vi "Stack Management.vi"(0 "Suck":bool) -> (1 "IsSucking?":bool, 2 "Full Stack (4 discs in)":bool)   [LabVIEW 2012]
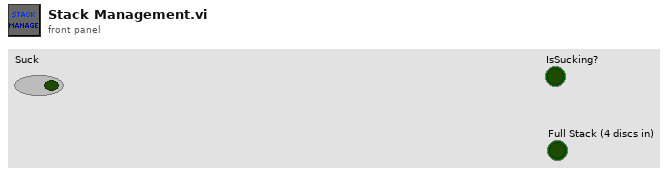
[diagram p1: front panel]
types:
  T1 = typedef "WPI_MotorControlDeviceRef.ctl" = cluster{"DeviceStatus":errorcluster, "Type":enum16{"PWM", "CAN"}, "PWM":cluster{"Digital Module":T2, "PWM Channel":T3, "DeadBand":T4}, "CAN":cluster{"Device Number":u8, "Control Mode":T5, "Semaphore":T6, "Max Vout":dbl}, "Invert":bool, "TransformRef":T7, "InvTransformRef":T7}
  T2 = typedef "FPGA_TypedefDigitalModule.ctl" = enum16{"Digital Module 1", "Digital Module 2"}
  T3 = typedef "FPGA_DIOPWMChannel.ctl" = enum8{"PWM 1", "PWM 2", "PWM 3", "PWM 4", "PWM 5", "PWM 6", "PWM 7", "PWM 8", "PWM 9", "PWM 10", "Invalid"}
  T4 = typedef "WPI_PWMDeadband.ctl" = cluster{"Name":string, "maxPositivePwm":i32, "minPositivePwm":i32, "centerPwm":i32, "maxNegativePwm":i32, "minNegativePwm":i32, "angularRange":u16}
  T5 = typedef "WPI_CANJaguar_ControlMode.ctl" = enum8{"Percent VBus", "Current", "Speed", "Position", "Voltage"}
  T6 = typedef "Semaphore RefNum" = refnum<k1>
  T7 = typedef "WPI_PWMTransform_ConPane.ctl" = refnum<vi>
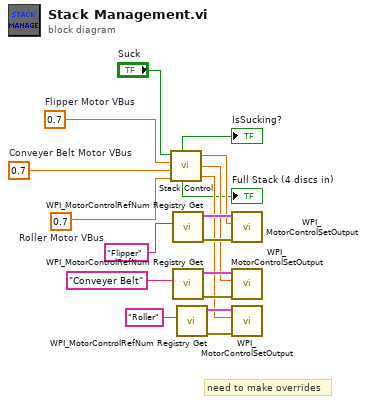
[diagram p0: block diagram]
diagram:
  w7 = 0.7  # Roller Motor VBus
  w8 = 0.7  # Conveyer Belt Motor VBus
  w9 = 0.7  # Flipper Motor VBus
  # "need to make overrides"
  n1 = call "Stack Control.vi"("Suck"="Suck", "Flipper Motor VBus"=w9, "Conveyer Belt Motor VBus"=w8, "Roller Motor VBus"=w7) -> ("IsSucking"=→"IsSucking?":bool, "Full Stack (4 discs in)"=→"Full Stack (4 discs in)":bool, "Flipper VBus out"=w2:dbl, "Conveyer Belt VBus out"=w3:dbl, "Roller VBus out"=w4:dbl)
  n2 = call <vilib>:"WPI_MotorControlRefNum Registry Get.vi"("refnum name"="Flipper") -> ("error out"=w12:errorcluster, "MotorControlDevRef"=w18:T1)  [unwired: 9 in]
  n3 = call <vilib>:"WPI_MotorControlRefNum Registry Get.vi"("refnum name"="Conveyer Belt") -> ("error out"=w11:errorcluster, "MotorControlDevRef"=w17:T1)  [unwired: 9 in]
  n4 = call <vilib>:"WPI_MotorControlRefNum Registry Get.vi"("refnum name"="Roller") -> ("error out"=w10:errorcluster, "MotorControlDevRef"=w16:T1)  [unwired: 9 in]
  n5 = call <vilib>:"WPI_MotorControlSetOutput.vi"("error in (no error)"=w12, "Output"=w2, "MotorControlDevRef"=w18) -> ()  [unwired: 6 in, 3 out]
  n6 = call <vilib>:"WPI_MotorControlSetOutput.vi"("error in (no error)"=w11, "Output"=w3, "MotorControlDevRef"=w17) -> ()  [unwired: 6 in, 3 out]
  n7 = call <vilib>:"WPI_MotorControlSetOutput.vi"("error in (no error)"=w10, "Output"=w4, "MotorControlDevRef"=w16) -> ()  [unwired: 6 in, 3 out]
